vi "Regl_nivel.vi"() -> ()   [LabVIEW 2010]
panel:
  out "u,y,r":cluster{"y":dbl, "u":dbl, "r-Set point":dbl}(graph)={"y"=4.981818181818582, "u"=4.98181818182085, "r-Set point"=4.9818181818181815}
  out "Comanda":dbl(slide)=4.981818181818582 scale=40.0..60.0
  out "Nivel":dbl(slide)=4.98181818182085 scale=40.0..60.0
  in  "Referinta":dbl(slide)=50.10909090909091 scale=40.0..60.0
  in  "Kd":dbl(slide)=0.10101010101010102 scale=0.0..0.5
  in  "Ki":dbl(slide)=0.9090909090909092 scale=0.0..2.0
  in  "Kp":dbl(slide)=0.4292929292929293 scale=0.0..2.5
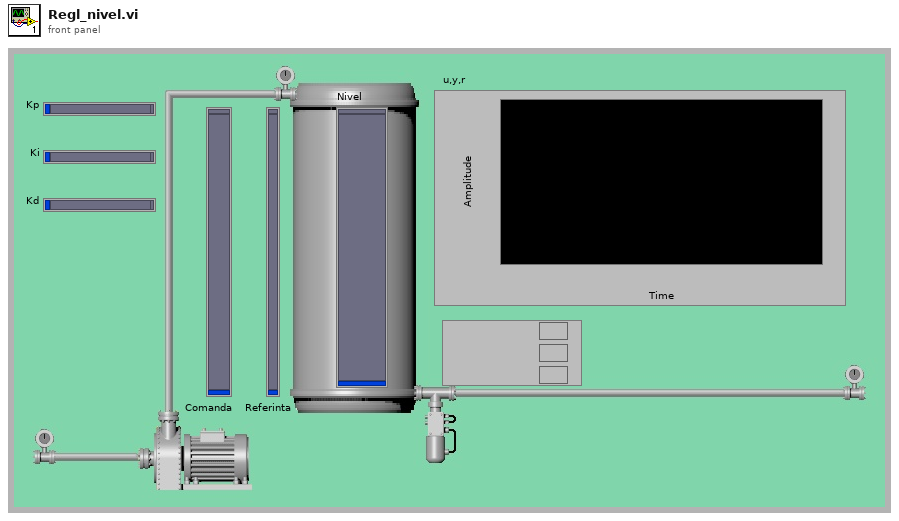
[diagram p1: front panel]
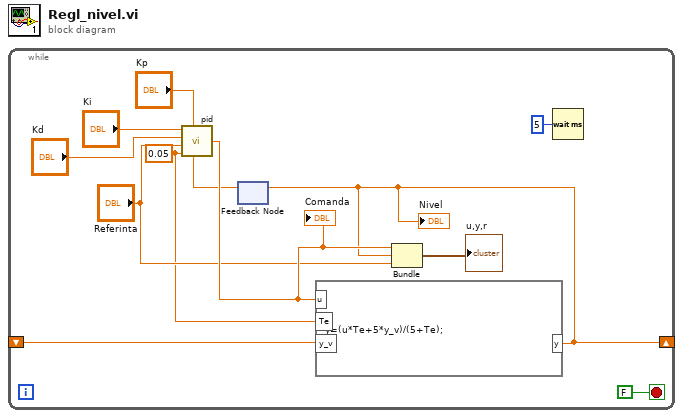
[diagram p0: block diagram]
diagram:
  n1 = while {
    shift-right: [w3] -> _
    shift-left: _ -> [w2]
    stop <- FALSE stop-if-true
    w5 = 0.05 ("Te")
    n2 = feedback #1() -> (w1:dbl)  [unwired: 1 in]
    n3 = call "pid.vi"("y"=w1, "Kp"="Kp", "Te"=w5, "r-Set point"="Referinta", "Kd"="Kd", "Ki"="Ki") -> ("u"=w8:dbl)
    "Comanda" <- w8
    n4 = formula code="y=(u*Te+5*y_v)/(5+Te);"("u"=w8, "Te"=w5, "y_v"=w2) -> ("y"=w3:dbl)
    "Nivel" <- w3
    n5 = feedback-in #1(w3) -> ()
    n6 = Bundle("u"=w8, "y"=w3, "Referinta"="Referinta") -> (→"u,y,r":cluster{"u":dbl, "y":dbl, "Referinta":dbl})  [unwired: 1 in]
    n7 = Wait (ms)(milliseconds to wait=u32 5) -> ()  [unwired: 1 out]
  }
